vi "merFISH_resume_tasks_list_TDMS.vi"(3 "error in":errorcluster, 4 "merFISH path":path=path "E:/") -> (0 "error out":errorcluster, 1 "refnum log file":refnum<file>)   [LabVIEW 2015]
uses:
  CONTROLS/Q_main_element.ctl
  GLOBAL/Global_MAIN.vi
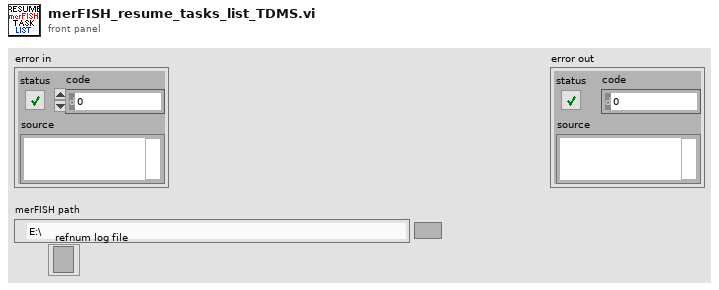
[diagram p1: front panel]
types:
  T1 = typedef "Q_main_element.ctl" = cluster{"variant":variant, "Instruction":enum16{"Main_idle", "Main_initialize", "Main_initialize_TDMS", "Main_initialize_Queue", "Main_error", "Main_DAQ_initialization_results", "Main_ASI_initialization_results", "Main_Piezo_initialization_results", "Main_Valve_initialization_results", "Main_Pump_initialization_results", "Main_CAMERA_initialization_results", "Main_DAQ_error", "Main_ASI_error", "Main_Piezo_error", "Main_CAMERA_error", "Main_Valve_error", "Main_Pump_error", "Main_start_acquiring", "Main_not_acquiring", "Main_acquiring", "Main_stop_acquiring", "Main_change_exposure", "Main_change_z_scan_parameters", "Main_define_ROI", "Main_read_kinetic_time", "Main_cooler", "Main_read_temperature", "Main_save_XY", "Main_load_XY", "Main_discard_XY", "Main_move_to_XY", "Main_measure_QPD", "Main_autofocus_calibration", "Main_save_PID", "Main_change_H_valve_position", "Main_two_way_valve", "Main_save_movie", "Main_init_single_scan", "Main_single_scan", "Main_stop_single_scan", "Main_merFISH_illumination_parameters", "Main_merFISH_buffer_probe_list", "Main_merFISH_injections_procedure", "Main_merFISH_save_setpoint", "Main_merFISH_init", "Main_merFISH_resume", "Main_merFISH_start_autofocus", "Main_merFISH_open_close_valve_merFISH", "Main_merFISH_open_close_valve_photobleaching", "Main_merFISH_hybridization", "Main_merFISH_move_to_ROI", "Main_merFISH_wait_stabilization", "Main_merFISH_scan", "Main_merFISH_photobleaching_injection", "Main_merFISH_photobleaching", "Main_merFISH_save", "Main_merFISH_send_email", "Main_merFISH_close", "Main_TL_define_parameters", "Main_TL_init", "Main_TL_start_autofocus", "Main_TL_move_to_ROI", "Main_TL_wait_for_stabilization", "Main_TL_scan", "Main_TL_wait_cycle_end", "Main_TL_close", "Main_STOP"}}
  T2 = enum16{"open", "replace", "create", "open or create", "replace or create", "replace or create with confirmation"}
  T3 = enum16{"open", "open or create", "create or replace", "create", "open (read-only)"}
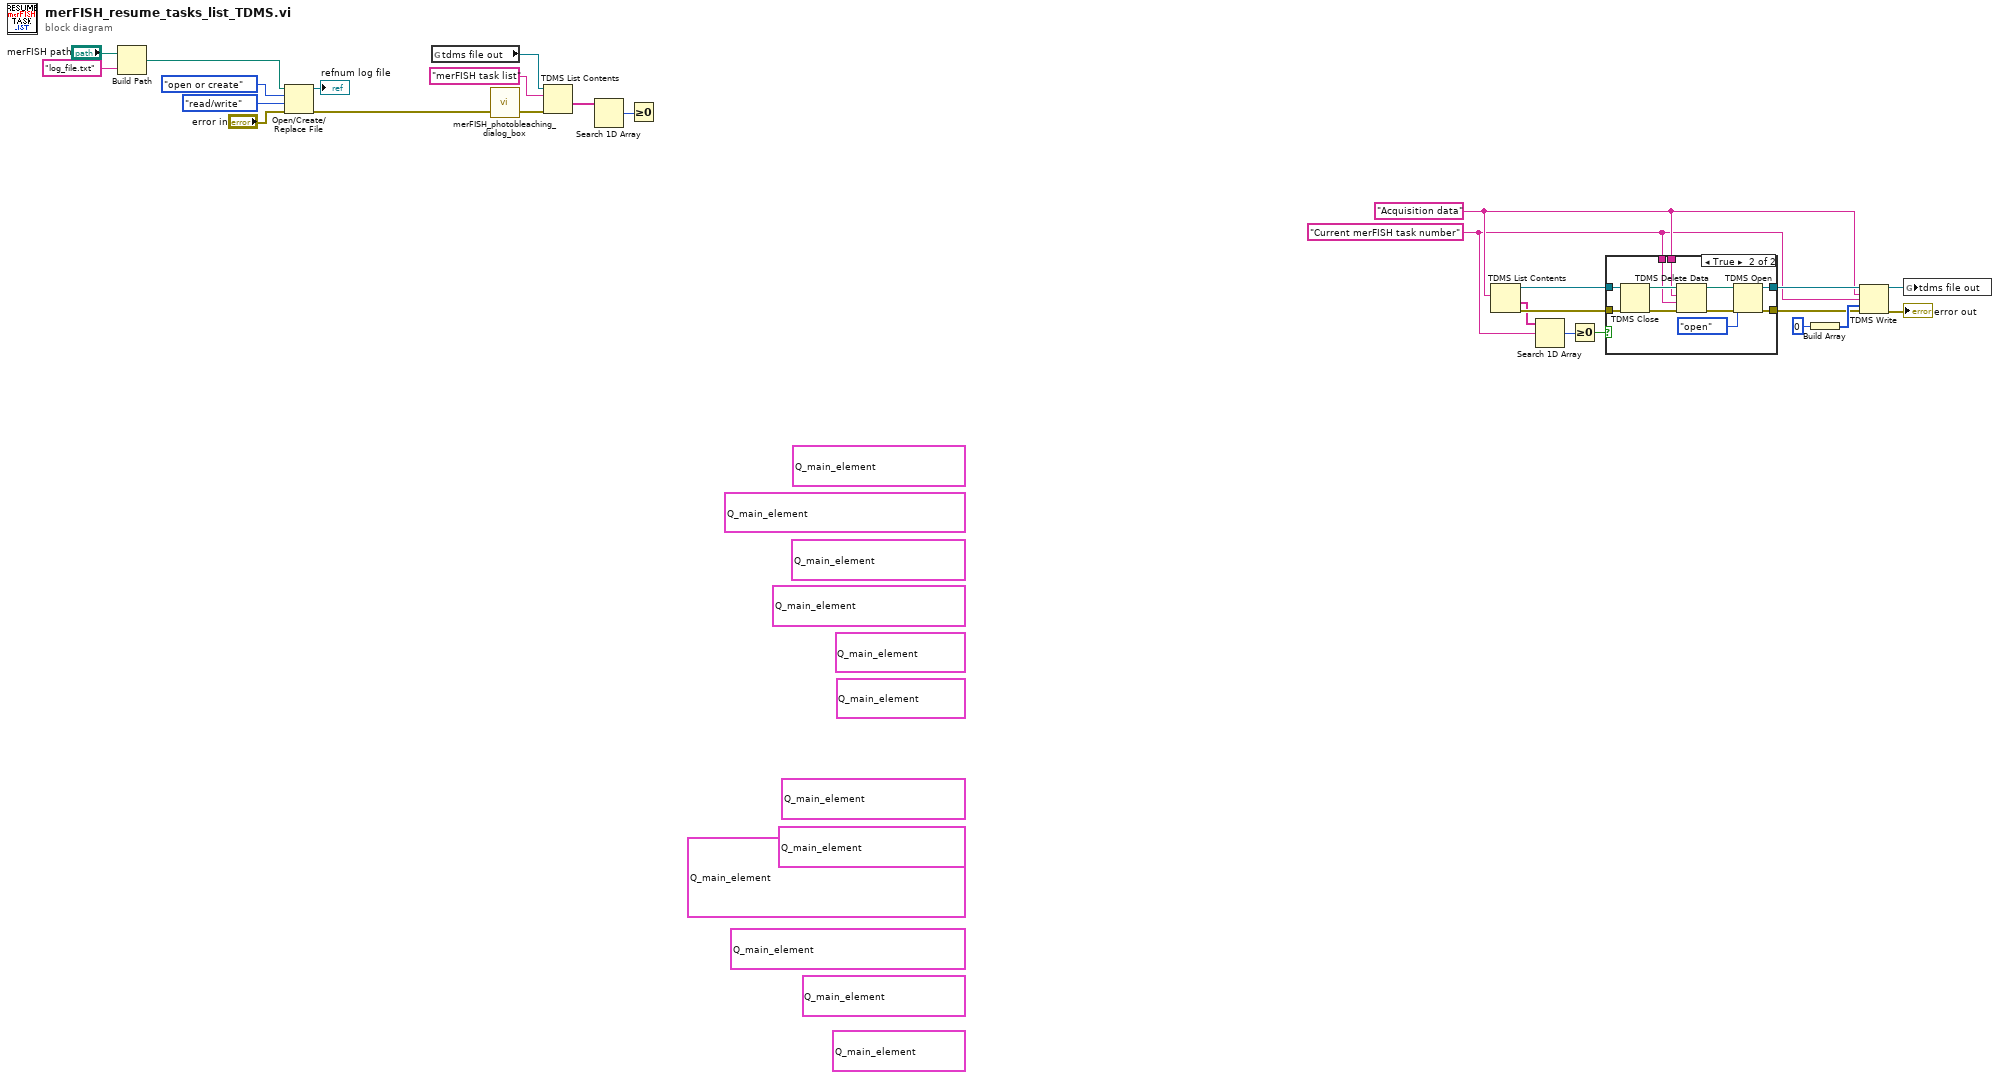
[diagram p0: block diagram]
diagram:
  w11 = "Current merFISH task number" ("group name in")
  w12 = "Acquisition data" ("group name in")
  w22 = T1 {"variant"=variant, "Instruction"=enum."Main_merFISH_open_close_valve_photobleaching"} ("element")
  w23 = T1 {"variant"=variant, "Instruction"=enum."Main_merFISH_send_email"} ("element")
  w31 = T1 {"variant"=variant, "Instruction"=enum."Main_merFISH_photobleaching_injection"} ("element")
  w32 = T1 {"variant"=variant, "Instruction"=enum."Main_merFISH_open_close_valve_merFISH"} ("element")
  w33 = T1 {"variant"=variant, "Instruction"=enum."Main_merFISH_hybridization"} ("element")
  w34 = T1 {"variant"=variant, "Instruction"=enum."Main_merFISH_close"} ("element")
  w35 = T1 {"variant"=variant, "Instruction"=enum."Main_merFISH_photobleaching"} ("element")
  w37 = T1 {"variant"=variant, "Instruction"=enum."Main_merFISH_save"} ("element")
  w38 = T1 {"variant"=variant, "Instruction"=enum."Main_merFISH_scan"} ("element")
  w39 = T1 {"variant"=variant, "Instruction"=enum."Main_merFISH_wait_stabilization"} ("element")
  w36 = T1 {"variant"=variant, "Instruction"=enum."Main_merFISH_start_autofocus"} ("element")
  w40 = T1 {"variant"=variant, "Instruction"=enum."Main_merFISH_move_to_ROI"} ("element")
  n1 = Build Path(base path="merFISH path", name or relative path="log_file.txt") -> (appended path=w28:path)
  n2 = Open/Create/Replace File(file path (use dialog)=w28, error in="error in", operation (0:open)=T2."open or create", access (0:read/write)=enum16{"read/write", "read-only", "write-only"}."read/write") -> (refnum out=→"refnum log file":refnum<file>, error out=w1:errorcluster)  [unwired: 2 in, 1 out]
  n3 = global read "Global_MAIN.vi" "tdms file out"() -> (w6:refnum<k34>)
  n4 = call "merFISH_photobleaching_dialog_box.vi"("error in"=w1) -> ("error out"=w5:errorcluster)  [unwired: 1 in, 1 out]
  n5 = TDMS List Contents(4:w5, 6:"merFISH task list" ("group name in (Untitled)"), 7:w6) -> (1:w2:string[])  [unwired: 3 out]
  n6 = Search 1D Array(1D array=w2) -> (index of element=w3:i32)  [unwired: 2 in]
  n7 = Greater Or Equal To 0?(x=w3) -> ()  [unwired: 1 out]
  n8 = TDMS List Contents(6:w12) -> (0:w20:errorcluster, 1:w17:string[], 3:w19:refnum<k34>, 4:w14:errorcluster, 7:w13:refnum<k34>)  [unwired: 1 out]
  n9 = Search 1D Array(1D array=w17, element=w11) -> (index of element=w18:i32)  [unwired: 1 in]
  n10 = Greater Or Equal To 0?(x=w18) -> (x >= 0?=w21:bool)
  n11 = case shown="True" w21 {
    tunnel: [w42 w50] -> w16
    tunnel: [w41 w49] -> w8
    tunnel: w19 -> [w42 w46]
    tunnel: w20 -> [w41 w45]
    tunnel: w11 -> [_ w44]
    tunnel: w12 -> [_ w43]
    frame False {
    }
    frame True {
      n12 = TDMS Close(8:w45, 11:w46) -> (0:w47:errorcluster, 3:w48:path)
      n13 = TDMS Delete Data(8:w47, 9:w44, 10:w43, 11:w48) -> (0:w52:errorcluster, 3:w53:path)  [unwired: 3 in]
      n14 = TDMS Open(8:w52, 10:T3."open" ("operation (0:open)"), 11:w53) -> (0:w49:errorcluster, 3:w50:refnum<k34>)  [unwired: 4 in]
    }
  }
  n15 = Build Array(u32 0) -> (w15:u32[])
  n16 = TDMS Write(0:w16, 5:w12, 7:w11, 9:w15, 11:w8) -> (4:w10:refnum<k34>, 15:→"error out":errorcluster)  [unwired: 1 in, 2 out]
  n17 = global write "Global_MAIN.vi" "tdms file out"(w10) -> ()
